vi "Verbal.vi"() -> ()   [LabVIEW 2018]
panel:
  in  "小平台X限位":dbl caption="小平台X轴限位/um" min=-8388607.0 max=8388607.0
  in  "UI状态":enum16{"UIEn", "UIDis"}(ring)
  out "上一次位置":i32[](array[numeric])
  out "xz0?":bool
  out "P3右":bool
  out "P2右":bool
  out "P1右":bool
  in  "pic_length":i32
  out "pz0?":bool
  out "py0?":bool
  out "px0?":bool
  in  "speed step":i32
  out "位置":dbl[][](array[numeric])
  in  "acc pic":i32
  in  "speed pic":i32
  in  "speed /rpm":dbl
  in  "Device Address":i32
  in  "Motor":i32
  out "DeviceKey":string
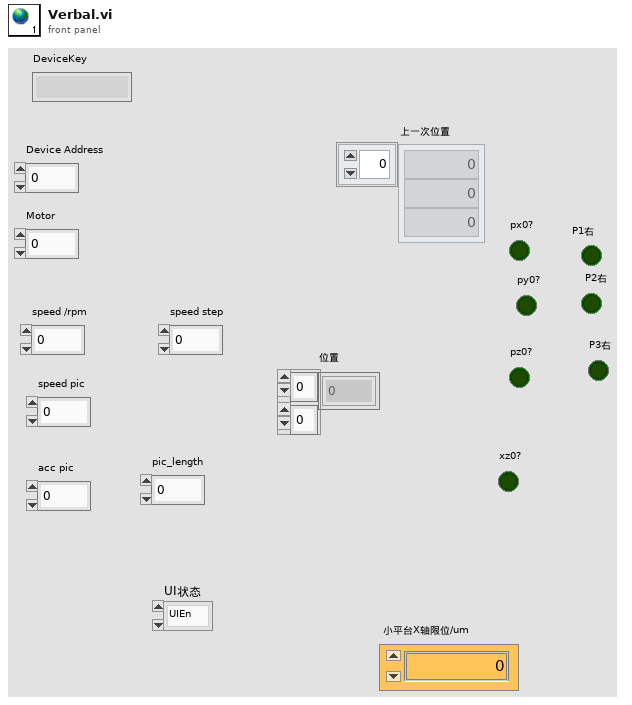
[diagram p1: front panel]
diagram:
